vi "ScanString.vi"(8 "error in (no error)":errorcluster, 10 "String":string, 11 "String D Element in":refnum<class "String D Element.lvclass">) -> (0 "error out":errorcluster, 3 "String D Element out":refnum<class "String D Element.lvclass">)   [LabVIEW 2020, in "D Datagrid Library.lvlib" / "String D Element.lvclass"]
uses:
  String D Element.lvclass
  String D Element.lvclass/String D Element.ctl
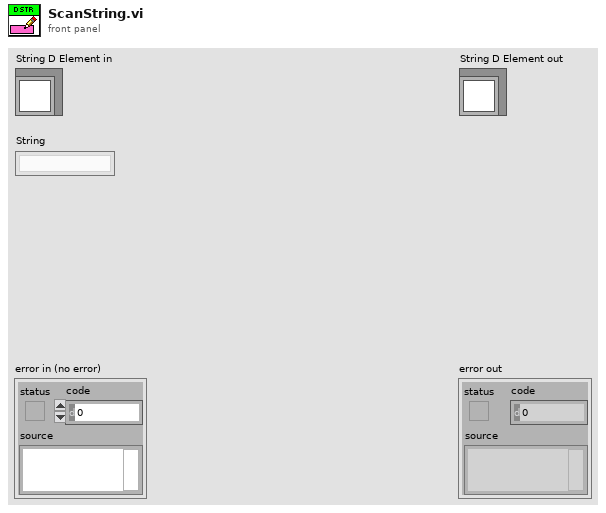
[diagram p1: front panel]
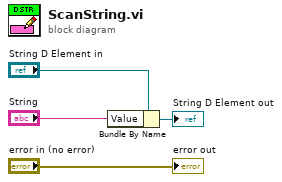
[diagram p0: block diagram]
diagram:
  n1 = Bundle By Name(cluster="String D Element in", "Value"="String") -> (→"String D Element out":refnum<class "String D Element.lvclass">)
  "error out" <- "error in (no error)"
